vi "TL behavior FWD obstacle avoidance.vi"(1 "Behavior\nVelocity":dbl=20.0, 2 "Activate?":bool=TRUE, 3 "Sensor":T1=[{"Name"="bow", "Angle"=10.0, "Distance"=0.0}, {"Name"="pbow", "Angle"=60.0, "Distance"=0.0}, {"Name"="port", "Angle"=0.0, "Distance"=0.0}, {"Name"="sbow", "Angle"=60.0, "Distance"=0.0}, {"Name"="starboard", "Angle"=0.0, "Distance"=0.0}]) -> (0 "Obs Avoid Array":dbl[](array[numeric]))   [LabVIEW 2014]
doc: "This vi uses the values from the Bow sensor to create an Obstacle Avoidance Array."
uses:
  sensorsSTD.ctl
panel:
  out "Waveform Graph":cluster{dbl, dbl, dbl[]}(graph)
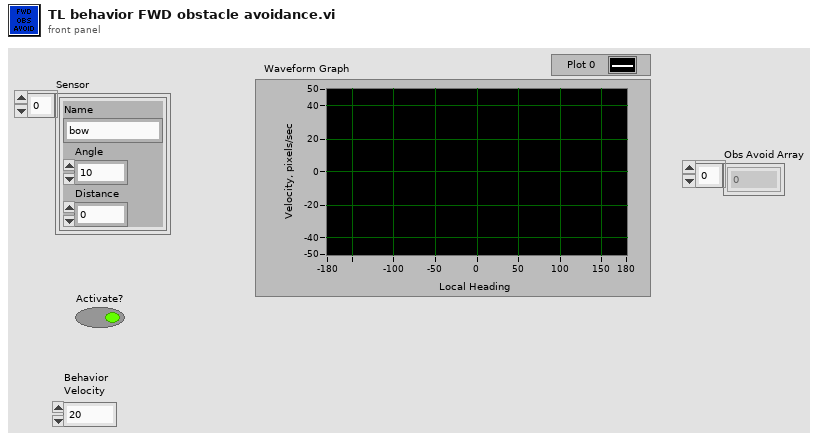
[diagram p1: front panel]
types:
  T1 = typedef "sensorsSTD.ctl" = cluster{"Name":string, "Angle":dbl, "Distance":dbl}[]
  T2 = cluster{"Name":string, "Angle":dbl, "Distance":dbl}
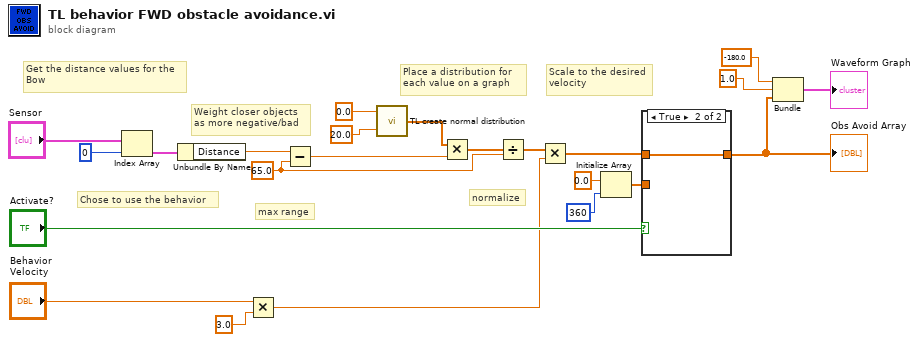
[diagram p0: block diagram]
diagram:
  w1 = 65.0 ("y")
  # "max range"
  # "Scale to the desired\nvelocity"
  # "Chose to use the behavior"
  # "Weight closer objects\nas more negative/bad"
  # "normalize"
  # "Place a distribution for \neach value on a graph"
  # "Get the distance values for the\nBow"
  n1 = Index Array(array="Sensor", index=0) -> (element=w21:T2)
  n2 = Unbundle By Name(w21) -> ("Distance"=w15:dbl)
  n3 = Multiply(x="Behavior\nVelocity", y=3.0) -> (x*y=w3:dbl)
  n4 = Subtract(x=w15, y=w1) -> (x-y=w14:dbl)
  n5 = call "TL create normal distribution.vi"("std (Normal)"=20.0, "mean"=0.0) -> ("ACT array"=w16:dbl[])
  n6 = Multiply(x=w16, y=w14) -> (x*y=w13:dbl[])
  n7 = Divide(x=w13, y=w1) -> (x/y=w7:dbl[])
  n8 = Multiply(x=w7, y=w3) -> (x*y=w6:dbl[])
  n9 = Initialize Array(0.0 ("element"), 360 ("dimension size")) -> (w9:dbl[])
  n10 = case shown="True" "Activate?" {
    tunnel: w6 -> [_ w25]
    tunnel: w9 -> [w24 _]
    tunnel: [w24 w25] -> w8
    frame False {
    }
    frame True {
    }
  }
  "Obs Avoid Array" <- w8
  n11 = Bundle(-180.0, 1.0, w8) -> (→"Waveform Graph":cluster{dbl, dbl, dbl[]})  [unwired: 1 in]
